vi "X Syringe Core.vi"() -> ()   [LabVIEW 2015]
uses:
  <vilib>/LabVIEW Targets/FPGA/cRIO/shared/nicrio_ModuleControls/nicrio_cRIO-9501_MicrostepRate.ctl
  <vilib>/LabVIEW Targets/FPGA/cRIO/shared/nicrio_ModuleControls/nicrio_cRIO-9501_CurrentReducPer.ctl
  Controls/Syringe State Enumerator.ctl
  <vilib>/ptbypt/NI_PtbyPt.lvlib
panel:
  in  "PID":cluster{"P":dbl, "I":dbl, "D":dbl}={"P"=1.0, "I"=0.5, "D"=0.5}
  in  "Current Reduction Delay":u16=100
  in  "Current Reduction Percentage":T1=enum."25 %"
  in  "Rated Phase Current":fxp<+/-,12,4>=0.3984375 format="%#_10g"
  in  "Microstepping Rate":T2
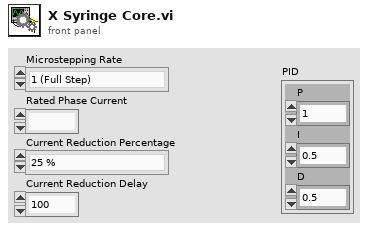
[diagram p1: front panel]
types:
  T1 = typedef "nicrio_cRIO-9501_CurrentReducPer.ctl" = enum8{"0 % (No Reduction)", "25 %", "50 %"}
  T2 = typedef "nicrio_cRIO-9501_MicrostepRate.ctl" = enum8{"1 (Full Step)", "2 (Half Step)", "4", "8", "16", "32", "64", "128", "256"}
  T3 = typedef "Syringe State Enumerator.ctl" = enum16{"Initialize", "Standby", "Enable", "Idle", "Prepare for Run", "Run", "Home", "Disable"}
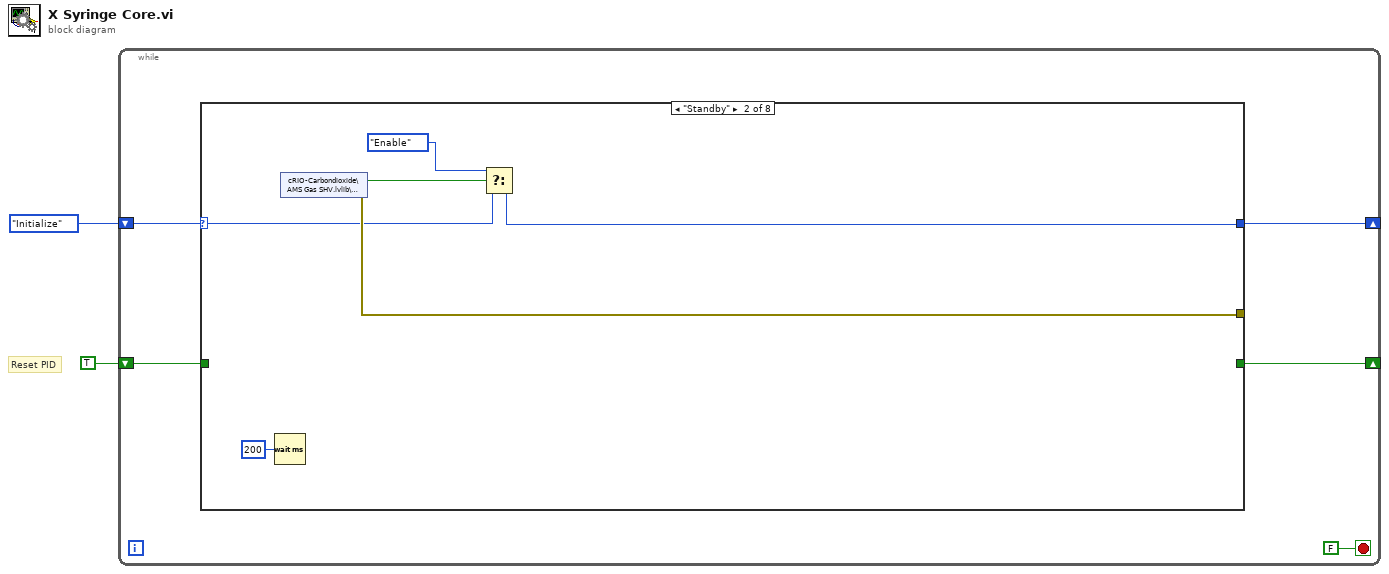
[diagram p0: block diagram]
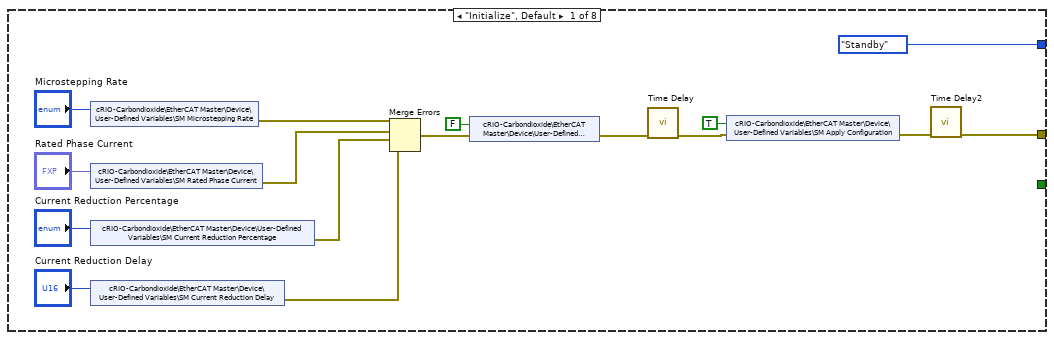
[diagram p2: hidden frame]
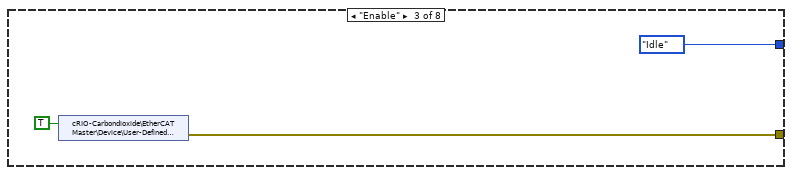
[diagram p3: hidden frame]
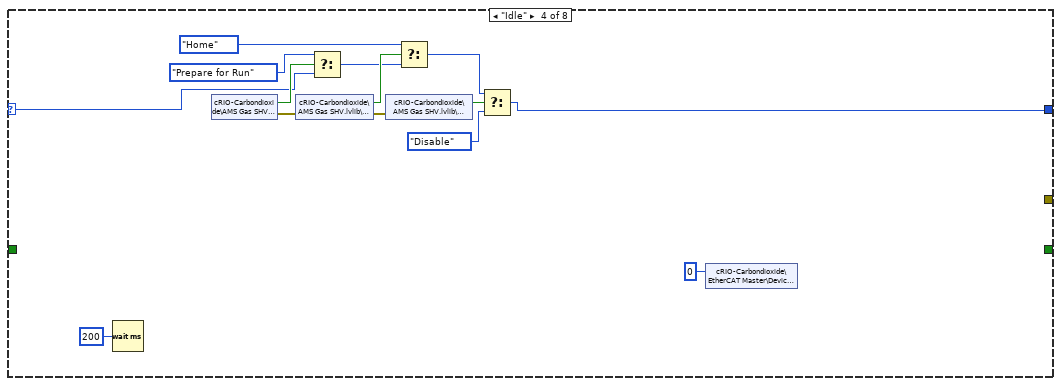
[diagram p4: hidden frame]
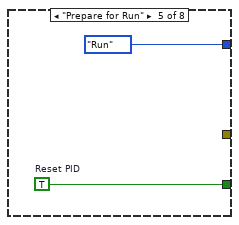
[diagram p5: hidden frame]
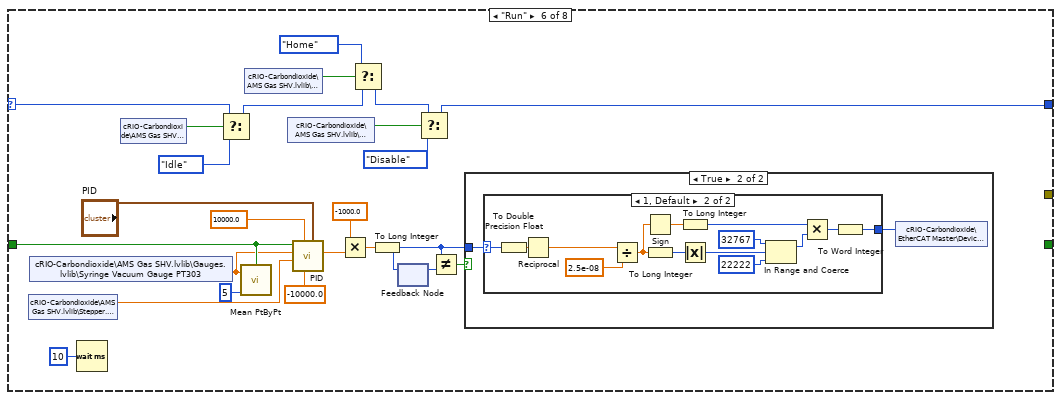
[diagram p6: hidden frame]
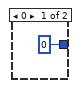
[diagram p8: hidden frame]
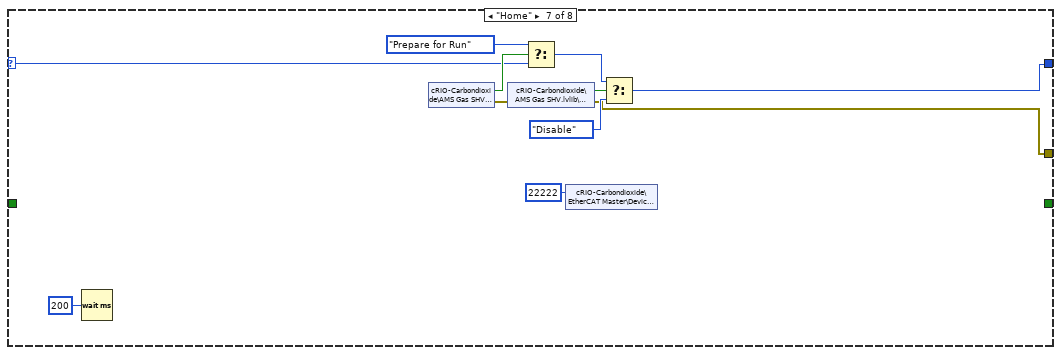
[diagram p9: hidden frame]
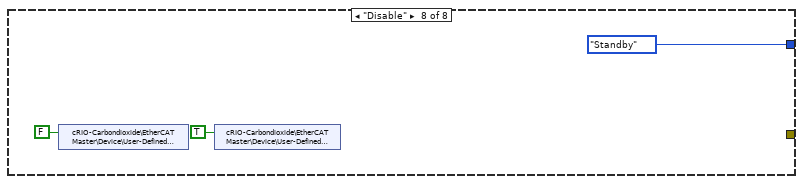
[diagram p10: hidden frame]
diagram:
  # "Reset PID"
  n1 = while {
    shift-right: [w6] -> _
    shift-left: Syringe_State_Enumerator."Initialize" -> [w5]
    shift-right: [w4] -> _
    shift-left: TRUE -> [w3]
    stop <- FALSE stop-if-true
    n2 = case shown="\"Standby\"" w5 {
      selector: w5 -> [_ w26 _ w42 _ w60 w94 _]
      tunnel: [Syringe_State_Enumerator."Standby" w25 Syringe_State_Enumerator."Idle" ("f") w39 Syringe_State_Enumerator."Run" ("f") w54 w97 Syringe_State_Enumerator."Standby" ("f")] -> w6
      tunnel: [w11 w27 w30 _ _ _ w91 _] -> _
      tunnel: [_ _ _ _ w48 _ _ _] -> w4
      tunnel: w3 -> [_ _ _ _ _ w50 _ _]
      frame "Initialize", Default {
        n3 = shared-variable "cRIO-Carbondioxide\\EtherCAT Master\\Device\\User-Defined Variables\\SM Microstepping Rate"("Microstepping Rate") -> (error out=w19:errorcluster)  [unwired: 1 in]
        n4 = shared-variable "cRIO-Carbondioxide\\EtherCAT Master\\Device\\User-Defined Variables\\SM Rated Phase Current"("Rated Phase Current") -> (error out=w16:errorcluster)  [unwired: 1 in]
        n5 = shared-variable "cRIO-Carbondioxide\\EtherCAT Master\\Device\\User-Defined Variables\\SM Current Reduction Percentage"("Current Reduction Percentage") -> (error out=w18:errorcluster)  [unwired: 1 in]
        n6 = shared-variable "cRIO-Carbondioxide\\EtherCAT Master\\Device\\User-Defined Variables\\SM Current Reduction Delay"("Current Reduction Delay") -> (error out=w17:errorcluster)  [unwired: 1 in]
        n7 = Merge Errors(w19, w16, w18, w17) -> (w9:errorcluster)
        n8 = shared-variable "cRIO-Carbondioxide\\EtherCAT Master\\Device\\User-Defined Variables\\SM Enable Drive"(FALSE ("Enable Drive"), error in=w9) -> (error out=w8:errorcluster)
        n9 = call "Time Delay"("error in (no error)"=w8) -> ("error out"=w13:errorcluster)  [unwired: 10 in]
        n10 = shared-variable "cRIO-Carbondioxide\\EtherCAT Master\\Device\\User-Defined Variables\\SM Apply Configuration"(TRUE ("Apply Configuration"), error in=w13) -> (error out=w12:errorcluster)
        n11 = call "Time Delay2"("error in (no error)"=w12) -> ("error out"=w11:errorcluster)  [unwired: 10 in]
      }
      frame "Standby" {
        n12 = Wait (ms)(milliseconds to wait=u32 200) -> ()  [unwired: 1 out]
        n13 = shared-variable "cRIO-Carbondioxide\\AMS Gas SHV.lvlib\\Stepper.lvlib\\Enabled"() -> (w28:bool, error out=w27:errorcluster)  [unwired: 1 in]
        n14 = Select(t=Syringe_State_Enumerator."Enable", s=w28, f=w26) -> (s? t:f=w25:T3)
      }
      frame "Enable" {
        n15 = shared-variable "cRIO-Carbondioxide\\EtherCAT Master\\Device\\User-Defined Variables\\SM Enable Drive"(TRUE ("Enable Drive")) -> (error out=w30:errorcluster)  [unwired: 1 in]
      }
      frame "Idle" {
        n16 = Wait (ms)(milliseconds to wait=u32 200) -> ()  [unwired: 1 out]
        n17 = shared-variable "cRIO-Carbondioxide\\AMS Gas SHV.lvlib\\Stepper.lvlib\\Run"() -> (w43:bool, error out=w37:errorcluster)  [unwired: 1 in]
        n18 = shared-variable "cRIO-Carbondioxide\\AMS Gas SHV.lvlib\\Stepper.lvlib\\Home"(error in=w37) -> (w46:bool, error out=w36:errorcluster)
        n19 = Select(t=Syringe_State_Enumerator."Prepare for Run", s=w43, f=w42) -> (s? t:f=w41:T3)
        n20 = shared-variable "cRIO-Carbondioxide\\AMS Gas SHV.lvlib\\Stepper.lvlib\\Enabled"(error in=w36) -> (w38:bool)  [unwired: 1 out]
        n21 = Select(t=Syringe_State_Enumerator."Home", s=w46, f=w41) -> (s? t:f=w40:T3)
        n22 = Select(t=w40, s=w38, f=Syringe_State_Enumerator."Disable") -> (s? t:f=w39:T3)
        n23 = shared-variable "cRIO-Carbondioxide\\EtherCAT Master\\Device\\User-Defined Variables\\SM Ticks"(i16 0 ("Ticks")) -> ()  [unwired: 1 in, 1 out]
      }
      frame "Prepare for Run" {
        w48 = TRUE  # Reset PID
      }
      frame "Run" {
        n24 = shared-variable "cRIO-Carbondioxide\\AMS Gas SHV.lvlib\\Stepper.lvlib\\Setpoint"() -> (w52:dbl)  [unwired: 1 in, 1 out]
        n25 = shared-variable "cRIO-Carbondioxide\\AMS Gas SHV.lvlib\\Gauges.lvlib\\Syringe Vacuum Gauge PT303"() -> (w49:dbl)  [unwired: 1 in, 1 out]
        n26 = Wait (ms)(milliseconds to wait=u32 10) -> ()  [unwired: 1 out]
        n27 = shared-variable "cRIO-Carbondioxide\\AMS Gas SHV.lvlib\\Stepper.lvlib\\Run"() -> (w63:bool)  [unwired: 1 in, 1 out]
        n28 = Select(t=w60, s=w63, f=Syringe_State_Enumerator."Idle") -> (s? t:f=w57:T3)
        n29 = call <vilib>:"Mean PtByPt.vi"("x"=w49, "sample length"=5, "initialize"=w50) -> ()  [unwired: 1 in, 2 out]
        n30 = shared-variable "cRIO-Carbondioxide\\AMS Gas SHV.lvlib\\Stepper.lvlib\\Home"() -> (w61:bool)  [unwired: 1 in, 1 out]
        n31 = shared-variable "cRIO-Carbondioxide\\AMS Gas SHV.lvlib\\Stepper.lvlib\\Enabled"() -> (w58:bool)  [unwired: 1 in, 1 out]
        n32 = call "PID.vi"("PID"="PID", "Lower Limit"=-10000.0, "Upper Limit (0,01)"=10000.0, "Setpoint (0,002)"=w52, "Process"=w49, "Reset"=w50) -> ("Output"=w65:dbl)  [unwired: 4 in, 1 out]
        n33 = Multiply(x=-1000.0, y=w65) -> (x*y=w68:dbl)
        n34 = Select(t=Syringe_State_Enumerator."Home", s=w61, f=w57) -> (s? t:f=w56:T3)
        n35 = To Long Integer(number=w68) -> (32bit integer=w66:i32)
        n36 = feedback #1() -> (w69:i32)  [unwired: 1 in]
        n37 = feedback-in #1(w66) -> ()
        n38 = Select(t=w56, s=w58, f=Syringe_State_Enumerator."Disable") -> (s? t:f=w54:T3)
        n39 = Not Equal?(x=w66, y=w69) -> (x != y?=w67:bool)
        n40 = case shown="True" w67 {
          tunnel: w66 -> [_ w74]
          frame False {
          }
          frame True {
            n41 = case shown="1, Default" w74 {
              selector: w74 -> [_ w88]
              tunnel: [i16 0 w76] -> w73
              frame 0 {
              }
              frame 1, Default {
                n42 = To Double Precision Float(number=w88) -> (double precision float=w79:dbl)
                n43 = Reciprocal(x=w79) -> (1/x=w78:dbl)
                n44 = Divide(x=w78, y=2.5e-08) -> (x/y=w89:dbl)
                n45 = Sign(1:w89) -> (0:w83:dbl)
                n46 = To Long Integer(number=w89) -> (32bit integer=w87:i32)
                n47 = To Long Integer(number=w83) -> (32bit integer=w82:i32)
                n48 = Absolute Value(x=w87) -> (abs(x)=w86:i32)
                n49 = In Range and Coerce(upper limit=32767, x=w86, lower limit=22222) -> (coerced(x)=w84:i32)  [unwired: 1 out]
                n50 = Multiply(x=w82, y=w84) -> (x*y=w81:i32)
                n51 = To Word Integer(number=w81) -> (16bit integer=w76:i16)
              }
            }
            n52 = shared-variable "cRIO-Carbondioxide\\EtherCAT Master\\Device\\User-Defined Variables\\SM Ticks"(w73) -> ()  [unwired: 1 in, 1 out]
          }
        }
      }
      frame "Home" {
        n53 = Wait (ms)(milliseconds to wait=u32 200) -> ()  [unwired: 1 out]
        n54 = shared-variable "cRIO-Carbondioxide\\AMS Gas SHV.lvlib\\Stepper.lvlib\\Run"() -> (w95:bool, error out=w92:errorcluster)  [unwired: 1 in]
        n55 = shared-variable "cRIO-Carbondioxide\\AMS Gas SHV.lvlib\\Stepper.lvlib\\Enabled"(error in=w92) -> (w99:bool, error out=w91:errorcluster)
        n56 = Select(t=Syringe_State_Enumerator."Prepare for Run", s=w95, f=w94) -> (s? t:f=w93:T3)
        n57 = shared-variable "cRIO-Carbondioxide\\EtherCAT Master\\Device\\User-Defined Variables\\SM Ticks"(i16 22222 ("Ticks")) -> ()  [unwired: 1 in, 1 out]
        n58 = Select(t=w93, s=w99, f=Syringe_State_Enumerator."Disable") -> (s? t:f=w97:T3)
      }
      frame "Disable" {
        n59 = shared-variable "cRIO-Carbondioxide\\EtherCAT Master\\Device\\User-Defined Variables\\SM Enable Drive"(FALSE ("Enable Drive")) -> ()  [unwired: 1 in, 1 out]
        n60 = shared-variable "cRIO-Carbondioxide\\EtherCAT Master\\Device\\User-Defined Variables\\SM Clear Faults"(TRUE ("Clear Faults")) -> ()  [unwired: 1 in, 1 out]
      }
    }
  }
